vi "Sting_umwandeln.vi"(0 "Lesepuffer":string, 11 "error in (no error)":errorcluster caption="Fehler (Eingang, kein Fehler)") -> (3 "Antwort gesamt":string, 4 "string array":string[](array[string]) caption="String-Array", 6 "Zahl array":dbl[](array[numeric]), 8 "Zahl als String array":string[](array[string]), 10 "original Cluster":T1, 14 "Array":string[](array[string]), 15 "error out":errorcluster caption="Fehler (Ausgang)")   [LabVIEW 2020, in "Linearisierung v2.lvlib" / "Gasteiler.lvlib" / "HovaCAL_Interface.lvlib" / "KGN.lvlib"]
uses:
  KGN.lvlib
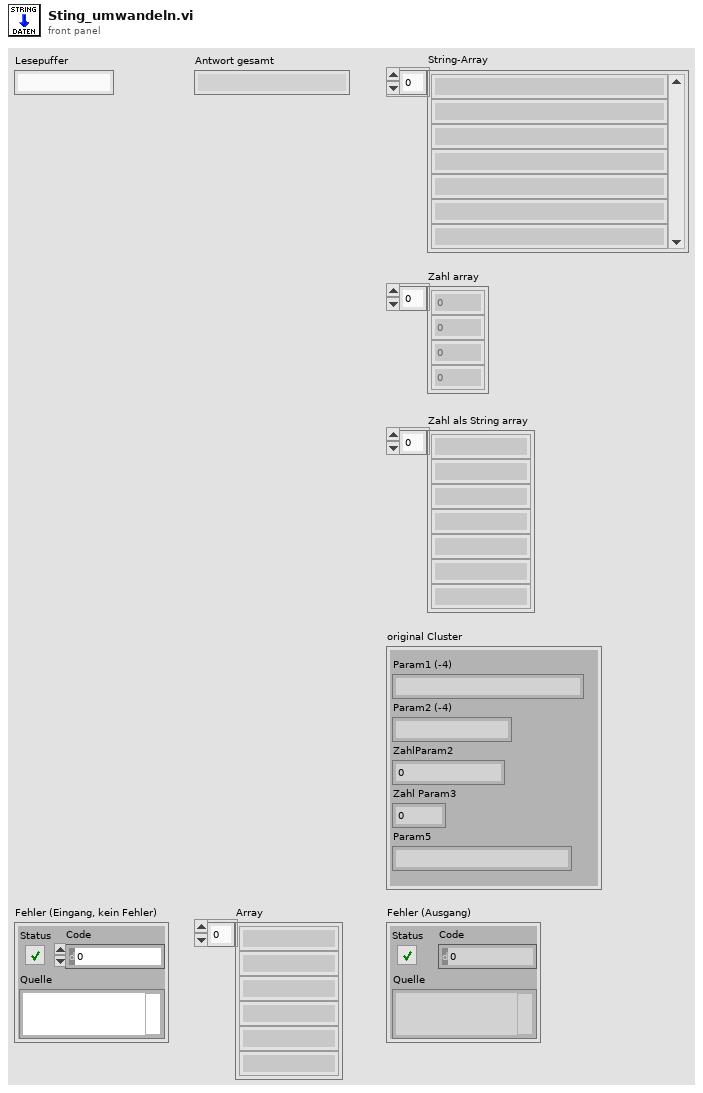
[diagram p1: front panel]
types:
  T1 = cluster{"Param1 (-4)":string, "Param2 (-4)":string, "ZahlParam2":dbl, "Zahl Param3":dbl, "Param5":string}
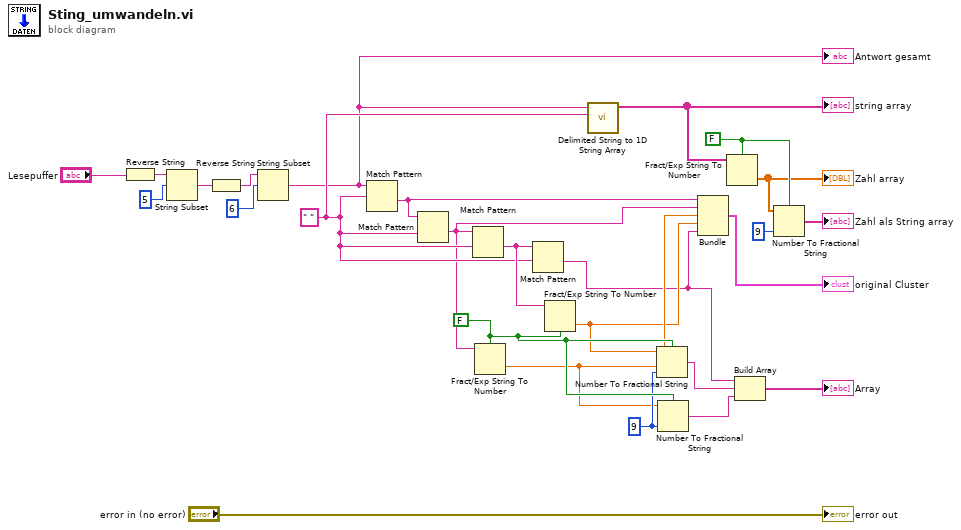
[diagram p0: block diagram]
diagram:
  w12 = FALSE ("Systemdezimalzeichen verwenden (T)")
  w16 = i16 9 ("Genauigkeit (6)")
  w17 = FALSE ("Systemdezimalzeichen verwenden (T)")
  w15 = " " ("Nach String/Zeichen suchen (-)")
  n1 = Reverse String(1:"Lesepuffer") -> (0:w22:string)
  n2 = String Subset(string=w22, offset (0)=5 ("Offset (0)")) -> (substring=w25:string)  [unwired: 1 in]
  n3 = Reverse String(1:w25) -> (0:w3:string)
  n4 = String Subset(string=w3, offset (0)=6 ("Offset (0)")) -> (substring=w2:string)  [unwired: 1 in]
  "Antwort gesamt" <- w2
  n5 = Match Pattern(string=w2, regular expression=w15) -> (after substring=w9:string)  [unwired: 1 in, 3 out]
  n6 = Match Pattern(string=w9, regular expression=w15) -> (after substring=w8:string)  [unwired: 1 in, 3 out]
  n7 = Match Pattern(string=w8, regular expression=w15) -> (after substring=w23:string)  [unwired: 1 in, 3 out]
  n8 = Fract/Exp String To Number(use system decimal point (T)=w17, string=w8) -> (number=w7:dbl)  [unwired: 2 in, 1 out]
  n9 = Match Pattern(string=w23, regular expression=w15) -> (after substring=w5:string)  [unwired: 1 in, 3 out]
  n10 = Fract/Exp String To Number(use system decimal point (T)=w17, string=w23) -> (number=w6:dbl)  [unwired: 2 in, 1 out]
  n11 = call <vilib>:"Delimited String to 1D String Array.vi"("delimiter"=w15, "delimited string"=w2) -> ("string array"=w14:string[])  [unwired: 9 in]
  "string array" <- w14
  n12 = Number To Fractional String(use system decimal point (T)=w17, number=w6, precision (6)=w16) -> (F-format string=w20:string)  [unwired: 1 in]
  n13 = Number To Fractional String(use system decimal point (T)=w17, number=w7, precision (6)=w16) -> (F-format string=w19:string)  [unwired: 1 in]
  n14 = Bundle(w9, w8, w7, w6, w5) -> (→"original Cluster":cluster{string, string, dbl, dbl, string})  [unwired: 1 in]
  n15 = Fract/Exp String To Number(use system decimal point (T)=w12, string=w14) -> (number=w11:dbl[])  [unwired: 2 in, 1 out]
  "Zahl array" <- w11
  n16 = Build Array(w5, w20, w19) -> (→"Array":string[])
  n17 = Number To Fractional String(use system decimal point (T)=w12, number=w11, precision (6)=i16 9 ("Genauigkeit (6)")) -> (F-format string=→"Zahl als String array":string[])  [unwired: 1 in]
  "error out" <- "error in (no error)"
